vi "SubVI_Complementary_Filter.vi"(9 "Gryo Displacement":dbl[](array[numeric]), 11 "Linear Acceleration":dbl[](array[numeric])) -> ()   [LabVIEW 2014]
uses:
  Globals_Real.vi
panel:
  in  "y":dbl=79.0 format="%#_13g"
  out "x < y?":bool
  out "Waveform Chart":dynamicdata(graph)
  out "X Disp":dbl
  out "x+y":dbl
  out "In Range?":bool
  out "Accel Magnitude":dbl
  # "Complentary FilTaH"
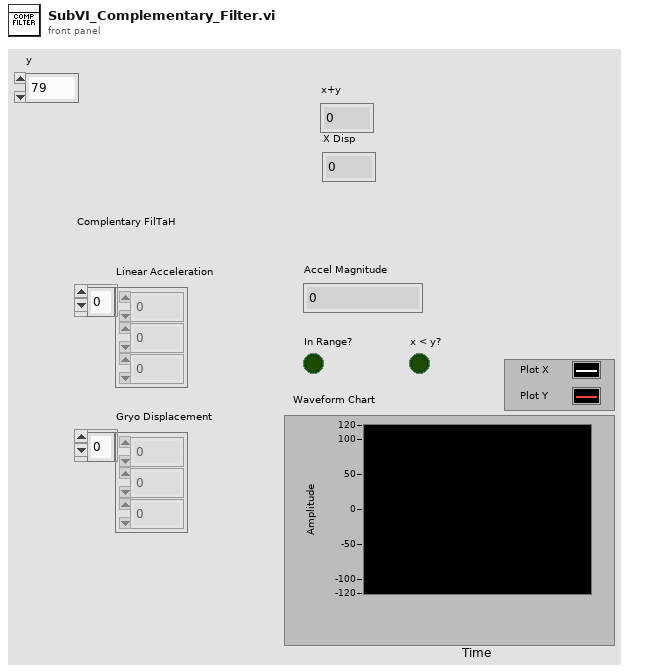
[diagram p1: front panel]
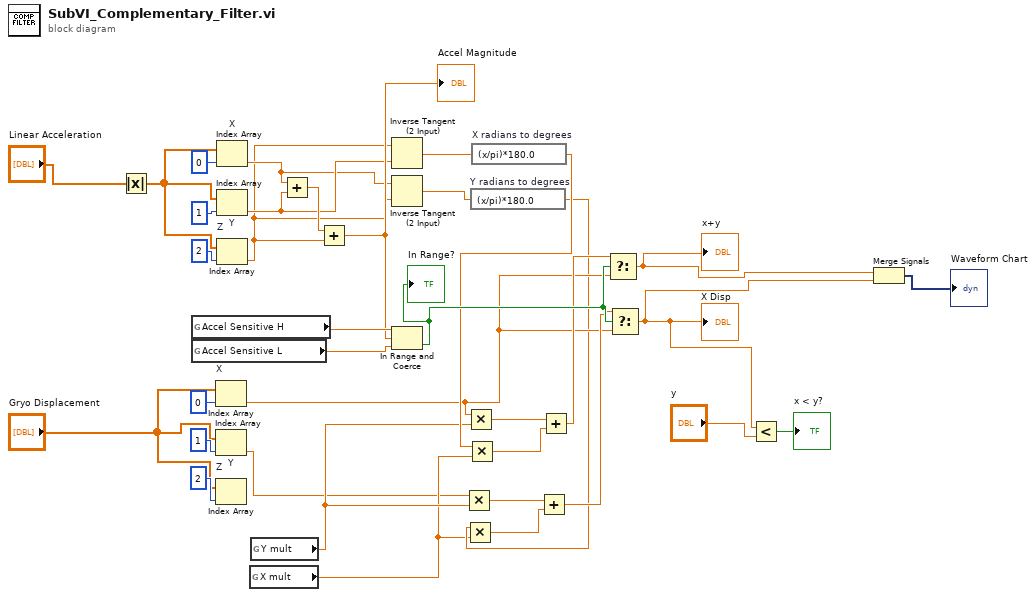
[diagram p0: block diagram]
diagram:
  n1 = Absolute Value(x="Linear Acceleration") -> (abs(x)=w31:dbl[])
  n2 = global read "Globals_Real.vi" "Accel Sensitive H"() -> (w30:dbl)
  n3 = global read "Globals_Real.vi" "Accel Sensitive L"() -> (w29:dbl)
  n4 = Index Array "X"(array="Gryo Displacement", index=0) -> (element=w13:dbl)
  n5 = Index Array "Y"(array="Gryo Displacement", index=1) -> (element=w7:dbl)
  n6 = Index Array "Z"(array="Gryo Displacement", index=2) -> ()  [unwired: 1 out]
  n7 = Index Array "X"(array=w31, index=0) -> (element=w2:dbl)
  n8 = Index Array "Y"(array=w31, index=1) -> (element=w3:dbl)
  n9 = Index Array "Z"(array=w31, index=2) -> (element=w1:dbl)
  n10 = global read "Globals_Real.vi" "X mult"() -> (w10:dbl)
  n11 = global read "Globals_Real.vi" "Y mult"() -> (w11:dbl)
  n12 = Add(x=w2, y=w3) -> (x+y=w33:dbl)
  n13 = Add(x=w33, y=w1) -> (x+y=w28:dbl)
  "Accel Magnitude" <- w28
  n14 = Inverse Tangent (2 Input)(1:w3, 2:w1) -> (0:w23:dbl)
  n15 = Inverse Tangent (2 Input)(1:w1, 2:w2) -> (0:w22:dbl)
  n16 = In Range and Coerce(upper limit=w30, x=w28, lower limit=w29) -> (In Range?=w21:bool)  [unwired: 1 out]
  "In Range?" <- w21
  n17 = Multiply(x=w7, y=w11) -> (x*y=w15:dbl)
  n18 = Multiply(x=w13, y=w11) -> (x*y=w20:dbl)
  n19 = expression code="(x/pi)*180.0" "Y radians to degrees"(w22) -> (w12:dbl)
  n20 = Multiply(x=w12, y=w10) -> (x*y=w16:dbl)
  n21 = expression code="(x/pi)*180.0" "X radians to degrees"(w23) -> (w17:dbl)
  n22 = Multiply(x=w17, y=w10) -> (x*y=w19:dbl)
  n23 = Add(x=w15, y=w16) -> (x+y=w14:dbl)
  n24 = Add(x=w20, y=w19) -> (x+y=w18:dbl)
  n25 = Select(t=w18, s=w21, f=w13) -> (s? t:f=w6:dbl)
  "x+y" <- w6
  n26 = Select(t=w14, s=w21, f=w13) -> (s? t:f=w5:dbl)
  "X Disp" <- w5
  n27 = Less?(x=w5, y="y") -> (x < y?=→"x < y?":bool)
  n28 = Merge Signals(w6, w5) -> (→"Waveform Chart":dynamicdata)
